vi "api_mqttInit.vi"(0 "client":string="LabVIEW_MQTT_Client", 5 "broker":T3={"address"="localhost", "port"=1883, "connTimeout"=2000, "writeTimeout"=2000, "readTimeout"=2000, "subTimeout"=30000}, 7 "connFlags":T2={"reserved"=FALSE, "clean session"=TRUE, "will flag"=TRUE, "willQOS"=enum."At most once", "will retain"=FALSE, "password"=FALSE, "user name"=FALSE}, 9 "User Info":T1={"User Name"="User", "Password"="password"}, 11 "error in (no error)":errorcluster) -> (15 "error out":errorcluster)   [LabVIEW 2013, in "mqtt.lvclass"]
uses:
  mqtt.lvclass
  mqttConfigFunction.ctl
  mqttTypedef/mqttBroker.ctl
  mqttTypedef/mqttConnectionFlags.ctl
  mqttTypedef/mqttWillInformation.ctl
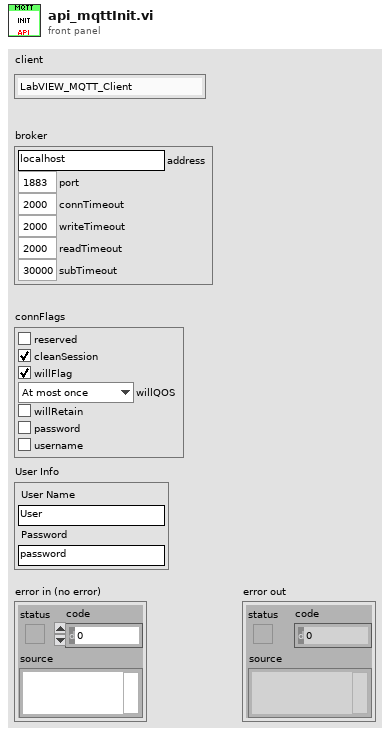
[diagram p1: front panel]
types:
  T1 = typedef "mqttWillInformation.ctl" = cluster{"User Name":string, "Password":string}
  T2 = typedef "mqttConnectionFlags.ctl" = cluster{"reserved":bool, "clean session":bool, "will flag":bool, "willQOS":enum8{"At most once", "At least once", "Exactly once", "Reserved"}, "will retain":bool, "password":bool, "user name":bool}
  T3 = typedef "mqttBroker.ctl" = cluster{"address":string, "port":u16, "connTimeout":i32, "writeTimeout":i32, "readTimeout":i32, "subTimeout":i32}
  T4 = typedef "mqtt.lvclass/mqttConfigFunction.ctl" = enum16{"init", "deinit", "set", "get"}
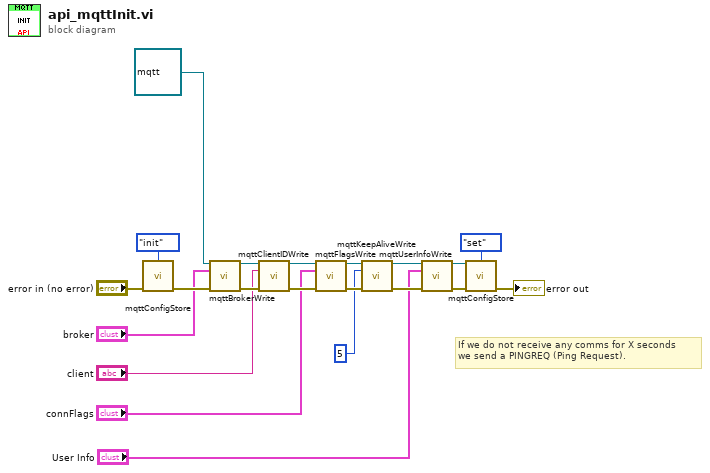
[diagram p0: block diagram]
diagram:
  # "If we do not receive any comms for X seconds\nwe send a PINGREQ (Ping Request)."
  n1 = call "mqttConfigStore.vi"("function"=mqttConfigFunction."init", "error in (no error)"="error in (no error)") -> ("error out"=w10:errorcluster)  [unwired: 12 in, 1 out]
  n2 = call "mqttBrokerWrite.vi"("mqtt in"=refnum<class "mqtt.lvclass"> refnum ("mqtt.lvclass"), "broker"="broker", "error in (no error)"=w10) -> ("mqtt out"=w21:refnum<class "mqtt.lvclass">, "error out"=w20:errorcluster)  [unwired: 11 in]
  n3 = call "mqttClientIDWrite.vi"("mqtt in"=w21, "clientID"="client", "error in (no error)"=w20) -> ("mqtt out"=w16:refnum<class "mqtt.lvclass">, "error out"=w15:errorcluster)  [unwired: 11 in]
  n4 = call "mqttFlagsWrite.vi"("mqtt in"=w16, "connFlags"="connFlags", "error in (no error)"=w15) -> ("mqtt out"=w18:refnum<class "mqtt.lvclass">, "error out"=w17:errorcluster)  [unwired: 11 in]
  n5 = call "mqttKeepAliveWrite.vi"("mqtt in"=w18, "keepAlive(sec)"=u16 5, "error in (no error)"=w17) -> ("mqtt out"=w5:refnum<class "mqtt.lvclass">, "error out"=w4:errorcluster)  [unwired: 11 in]
  n6 = call "mqttUserInfoWrite.vi"("mqtt in"=w5, "User Info"="User Info", "error in (no error)"=w4) -> ("mqtt out"=w2:refnum<class "mqtt.lvclass">, "error out"=w1:errorcluster)  [unwired: 11 in]
  n7 = call "mqttConfigStore.vi"("mqtt.lvclass in"=w2, "function"=mqttConfigFunction."set", "error in (no error)"=w1) -> ("error out"=→"error out":errorcluster)  [unwired: 11 in, 1 out]
